vi "Int16Scale_mV_1DArray.vi"(1 "Max Voltage":dbl, 2 "Int16Array":i16[](array[numeric])) -> (0 "Scaled mV Array":sgl[](array[numeric]))   [LabVIEW 2018]
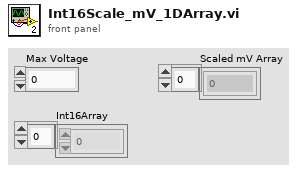
[diagram p1: front panel]
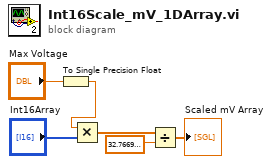
[diagram p0: block diagram]
diagram:
  n1 = To Single Precision Float(number="Max Voltage") -> (single precision float=w1:sgl)
  n2 = Multiply(x=w1, y="Int16Array") -> (x*y=w5:sgl[])
  n3 = Divide(x=w5, y=sgl 32.767) -> (x/y=→"Scaled mV Array":sgl[])
